vi "FT_Read_Byte_Data.vi"(0 "Handle":u32, 1 "Bytes To Read":u32) -> (2 "Handle":u32, 3 "Read Data":u8[](array[numeric]), 4 "FT_Status":u32, 5 "Bytes Read":u32)   [LabVIEW 2011]
uses:
  FTD2XX.dll
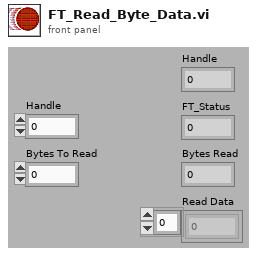
[diagram p1: front panel]
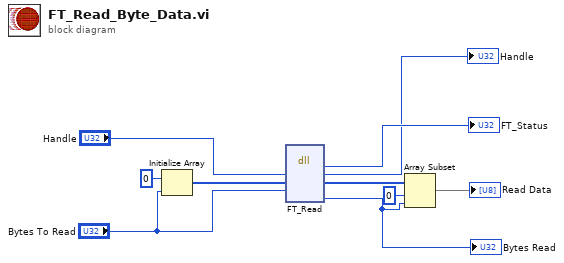
[diagram p0: block diagram]
diagram:
  n1 = Initialize Array(u8 0 ("element"), "Bytes To Read") -> (w8:u8[])
  n2 = dll-call lib="D:/WORK/LabView/#Avesta/D2XX_Functions_7.0/FTD2XX.dll" fn="FT_Read"("Handle"="Handle", "Buffer"=w8, "BytesToRead"="Bytes To Read") -> ("FT_Status"=→"FT_Status":u32, "Handle"=→"Handle":u32, "Buffer"=w5:u8[], "BytesReturned"=w3:u32)  [unwired: 4 in, 3 out]
  "Bytes Read" <- w3
  n3 = Array Subset(array=w5, index=0, length=w3) -> (→"Read Data":u8[])
